vi "Finish Command.vi"(8 "error in (no error)":errorcluster, 11 "Command in":refnum<class "Command Actor.lvclass">) -> (0 "error out":errorcluster, 3 "Command out":refnum<class "Command Actor.lvclass">)   [LabVIEW 2014, in "Robot Actor Framework.lvlib" / "Command Actor.lvlib" / "Command Actor.lvclass"]
uses:
  Command Actor.lvclass
  Command States.ctl
  <vilib>/ActorFramework/Message Enqueuer/Message Priority.ctl
  Command Actor.lvclass/Command Actor.ctl
  <vilib>/ActorFramework/Actor/Actor.lvclass/Actor.ctl
  Command Processor Actor/Command Processor Actor Messages/Command Finished Msg/Command Finished Msg.lvclass/Command Finished Msg.ctl
  <vilib>/ActorFramework/Message Enqueuer/Message Enqueuer.lvclass/Message Enqueuer.ctl
  <vilib>/ActorFramework/Message Enqueuer/Enqueue.vi
  <vilib>/ActorFramework/Message Priority Queue/Priority Enqueue.vi
  Command Processor Actor/Command Processor Actor Messages/Command Finished Msg/Command Finished Msg.lvclass
  <vilib>/ActorFramework/Actor/Actor.lvclass
  <vilib>/ActorFramework/Message Enqueuer/Message Enqueuer.lvclass
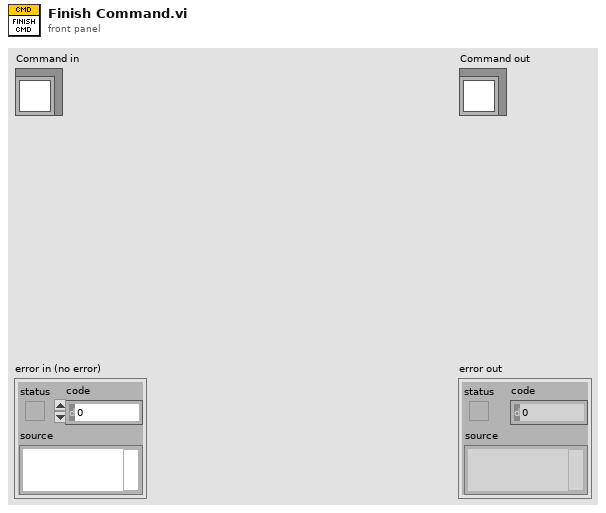
[diagram p1: front panel]
types:
  T1 = typedef "Actor Framework.lvlib/Message Enqueuer.lvclass/Message Priority.ctl" = enum16{"Low", "Normal", "High"}
  T2 = enum16{"Critical", "Error", "Warning", "Informational", "Debug"}
  T3 = typedef "Robot Actor Framework.lvlib/Command Actor.lvlib/Command Actor.lvclass/Command States.ctl" = enum16{"Unknown", "Started", "Stopped", "Finished"}
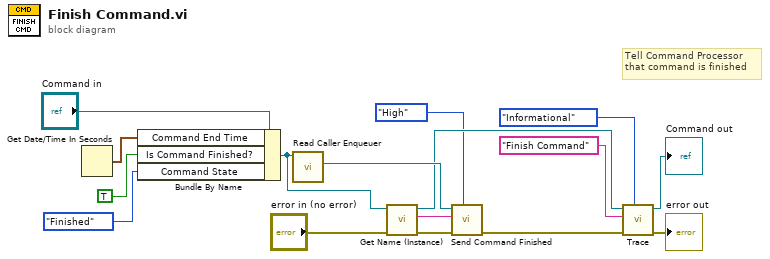
[diagram p0: block diagram]
diagram:
  # "Tell Command Processor\nthat command is finished"
  n1 = Get Date/Time In Seconds() -> (seconds since 1Jan1904=w14:timestamp)
  n2 = Bundle By Name(cluster="Command in", "Command End Time"=w14, "Is Command Finished?"=TRUE, "Command State"=Command_States."Finished") -> (w6:refnum<class "Command Actor.lvclass">)
  n3 = call <vilib>:"Read Caller Enqueuer.vi"("Actor"=w6) -> ("Caller Enqueuer"=w15:refnum<class "Message Enqueuer.lvclass">)  [unwired: 10 in]
  n4 = call-dynamic "Get Name (Instance).vi"("error in (no error)"="error in (no error)", "Command Actor in"=w6) -> ("error out"=w1:errorcluster, "Name (Instance)"=w4:string, "Command Actor out"=w5:refnum<class "Command Actor.lvclass">)  [unwired: 7 in]
  n5 = call "Send Command Finished.vi"("Message Priority (Normal)"=Message_Priority."High", "error in (no error)"=w1, "Command Name (Instance)"=w4, "Message Enqueuer"=w15) -> ("error out"=w10:errorcluster)  [unwired: 6 in, 1 out]
  n6 = call-dynamic "Trace.vi"("Trace Level"=T2."Informational", "error in (no error)"=w10, "Command Action"="Finish Command" ("Trace Message"), "Command Actor in"=w5) -> ("error out"=→"error out":errorcluster, "Command Actor out"=→"Command out":refnum<class "Command Actor.lvclass">)  [unwired: 6 in]
